vi "MidbrainBehaviorEngine.vi"(11 "ForebrainCom":T2) -> (0 "BehaviorInhibit":T1, 3 "VelCom":dbl)   [LabVIEW 2010]
doc: "This sub VI takes the commanded mission velocity and robot behavior from the Forebrain and activates the appropriate Midbrain subbehaviors to cary it out."
panel:
  # "This subVI takes the current desired robot\nvelocity andoverall  behavior from the Forebrain\nand activates the appropriate Midbrain sub-behaviors\nto carry it out"
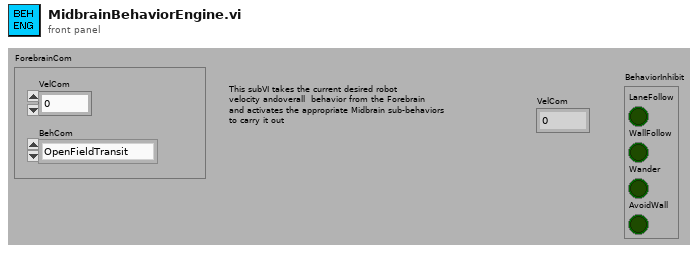
[diagram p1: front panel]
types:
  T1 = cluster{"AvoidWall":bool, "Wander":bool, "WallFollow":bool, "LaneFollow":bool}
  T2 = cluster{"VelCom":dbl, "BehCom":enum16{"OpenFieldTransit", "WallFollow", "LaneFollow", "ManualMode"}}
  T3 = enum16{"OpenFieldTransit", "WallFollow", "LaneFollow", "ManualMode"}
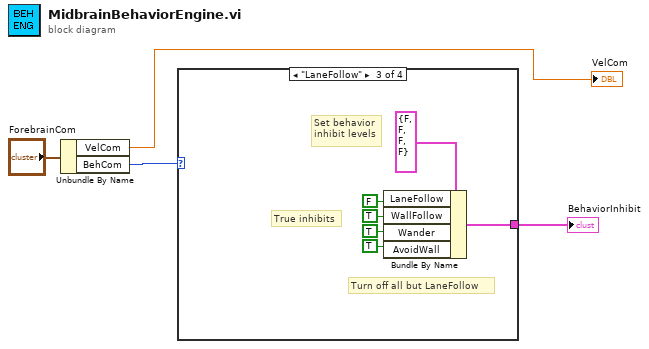
[diagram p0: block diagram]
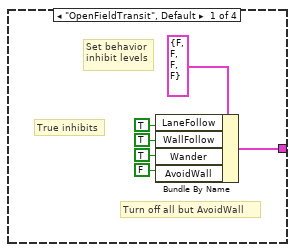
[diagram p2: hidden frame]
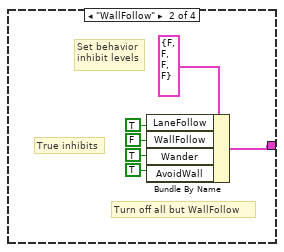
[diagram p3: hidden frame]
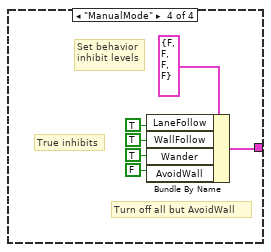
[diagram p4: hidden frame]
diagram:
  n1 = Unbundle By Name("ForebrainCom") -> ("VelCom"=→"VelCom":dbl, "BehCom"=w2:T3)
  n2 = case shown="\"LaneFollow\"" w2 {
    tunnel: [w9 w11 w17 w23] -> w1
    frame "OpenFieldTransit", Default {
      # "True inhibits"
      # "Set behavior\ninhibit levels"
      # "Turn off all but AvoidWall"
      n3 = Bundle By Name(cluster=T1 {"AvoidWall"=FALSE, "Wander"=FALSE, "WallFollow"=FALSE, "LaneFollow"=FALSE} ("BehaviorInhibit"), "LaneFollow"=TRUE, "WallFollow"=TRUE, "Wander"=TRUE, "AvoidWall"=FALSE) -> (w9:T1)
    }
    frame "WallFollow" {
      # "True inhibits"
      # "Set behavior\ninhibit levels"
      # "Turn off all but WallFollow"
      n4 = Bundle By Name(cluster=T1 {"AvoidWall"=FALSE, "Wander"=FALSE, "WallFollow"=FALSE, "LaneFollow"=FALSE} ("BehaviorInhibit"), "LaneFollow"=TRUE, "WallFollow"=FALSE, "Wander"=TRUE, "AvoidWall"=TRUE) -> (w11:T1)
    }
    frame "LaneFollow" {
      # "True inhibits"
      # "Set behavior\ninhibit levels"
      # "Turn off all but LaneFollow"
      n5 = Bundle By Name(cluster=T1 {"AvoidWall"=FALSE, "Wander"=FALSE, "WallFollow"=FALSE, "LaneFollow"=FALSE} ("BehaviorInhibit"), "LaneFollow"=FALSE, "WallFollow"=TRUE, "Wander"=TRUE, "AvoidWall"=TRUE) -> (w17:T1)
    }
    frame "ManualMode" {
      # "True inhibits"
      # "Set behavior\ninhibit levels"
      # "Turn off all but AvoidWall"
      n6 = Bundle By Name(cluster=T1 {"AvoidWall"=FALSE, "Wander"=FALSE, "WallFollow"=FALSE, "LaneFollow"=FALSE} ("BehaviorInhibit"), "LaneFollow"=TRUE, "WallFollow"=TRUE, "Wander"=TRUE, "AvoidWall"=FALSE) -> (w23:T1)
    }
  }
  "BehaviorInhibit" <- w1
